vi "Read Position Ref.vi"(8 "error in (no error)":errorcluster, 11 "Transform Ref in":refnum<vi>) -> (0 "error out":errorcluster, 2 "Position out":refnum<class "Vector2.lvclass">, 3 "Transform Ref out":refnum<vi>)   [LabVIEW 2022 SP3, in "Transform.lvclass"]
uses:
  Transform.lvclass
  Math/Vector2/Vector2.lvclass
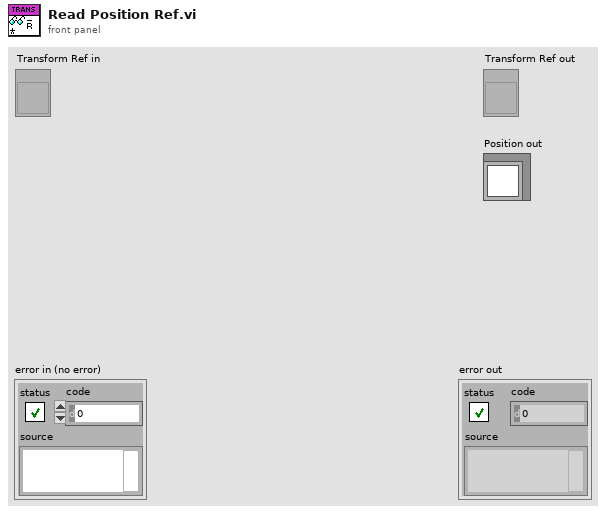
[diagram p1: front panel]
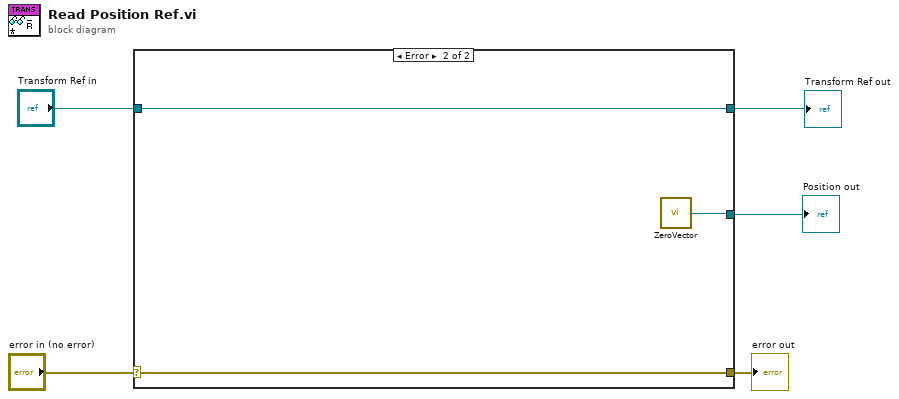
[diagram p0: block diagram]
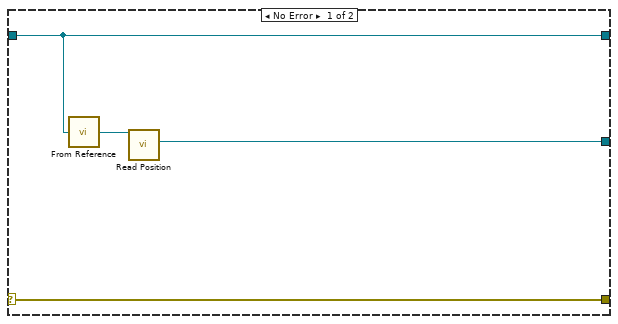
[diagram p2: hidden frame]
diagram:
  n1 = case shown="Error" "error in (no error)" {
    selector: "error in (no error)" -> [w9 w12]
    tunnel: [w9 w12] -> w4
    tunnel: [w8 w11] -> w2
    tunnel: "Transform Ref in" -> [w8 w11]
    tunnel: [w6 w10] -> w1
    frame No Error {
      n2 = call "From Reference.vi"("Transform Ref in"=w8) -> ("Transform out"=w7:refnum<class "Transform.lvclass">)
      n3 = call "Read Position.vi"("Transform in"=w7) -> ("Position out"=w6:refnum<class "Vector2.lvclass">)  [unwired: 8 in, 2 out]
    }
    frame Error {
      n4 = call "ZeroVector.vi"() -> ("Zero Vector"=w10:refnum<class "Vector2.lvclass">)
    }
  }
  "error out" <- w4
  "Transform Ref out" <- w2
  "Position out" <- w1
